vi "Read fit presets.vi"(0 "Config file in":T1, 11 "error in (no error)":errorcluster) -> (4 "Config file out":T1, 6 "Fit parameters":T3={"A"=0.572086, "S"=0.0835606, "M1"=140.286, "M2"=140.486}, 8 "Physical constants":T2={"T1e (s)"=0.03, "T1n (s)"=1500.0}, 10 "C":dbl, 14 "Key not found?":bool, 15 "error out":errorcluster)   [LabVIEW 2015]
uses:
  fit_parameters.ctl
  physical_constants.ctl
  <vilib>/Utility/config.llb/Config Data RefNum.ctl
  <vilib>/Utility/config.llb/Read Key (Double).vi
  <vilib>/Utility/config.llb/NI_LVConfig.lvlib
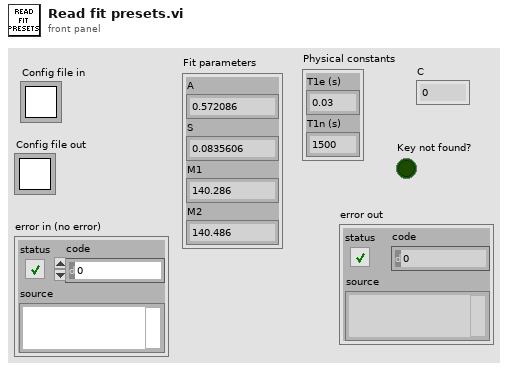
[diagram p1: front panel]
types:
  T1 = typedef "NI_LVConfig.lvlib/Config Data RefNum.ctl" = refnum<k1>
  T2 = typedef "physical_constants.ctl" = cluster{"T1e (s)":dbl, "T1n (s)":dbl}
  T3 = typedef "fit_parameters.ctl" = cluster{"A":dbl, "S":dbl, "M1":dbl, "M2":dbl}
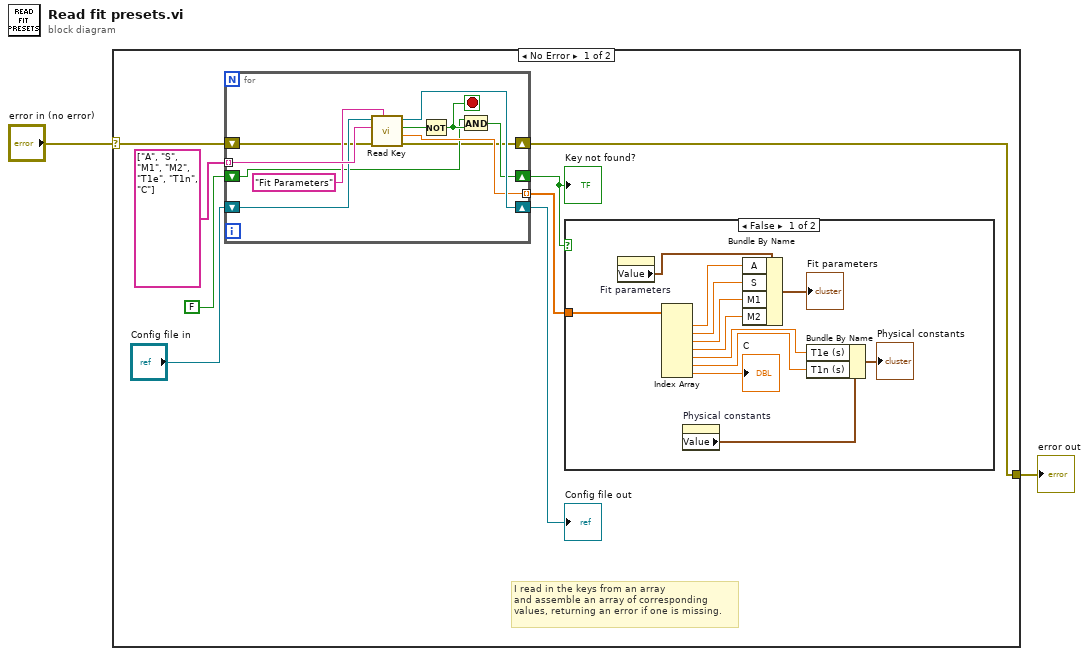
[diagram p0: block diagram]
diagram:
  n1 = case shown="No Error" "error in (no error)" {
    selector: "error in (no error)" -> [w4 w34]
    tunnel: [w3 w34] -> w1
    frame No Error {
      # "I read in the keys from an array\nand assemble an array of corresponding\nvalues, returning an error if one is missing."
      n2 = for {
        tunnel: string[] ["A", "S", "M1", "M2", "T1e", "T1n", "C"] -> [w33] mode=indexing
        shift-right: [w29] -> w5
        shift-left: "Config file in" -> [w30]
        tunnel: [w28] -> w9 mode=indexing
        shift-right: [w27] -> w7
        shift-left: FALSE -> [w25]
        shift-right: [w23] -> w3
        shift-left: w4 -> [w24]
        stop <- w26 stop-if-true
        n3 = call-poly <vilib>:"Read Key.vi"("section"="Fit Parameters", "error in (no error)"=w24, "key"=w33, "refnum"=w30) -> ("error out"=w23:errorcluster, "value"=w28:dbl, "found?"=w31:bool, "refnum out"=w29:T1)  [unwired: 4 in]
        n4 = Not(x=w31) -> (.not. x?=w26:bool)
        n5 = And(x=w25, y=w26) -> (x .and. y?=w27:bool)
      }
      "Key not found?" <- w7
      "Config file out" <- w5
      n6 = case shown="False" w7 {
        tunnel: w9 -> [w22 _]
        frame False {
          n7 = property on="Fit parameters" class="Clust (strict)"() -> ("Value"=w21:T3)  [unwired: 2 in, 2 out]
          n8 = Index Array(array=w22) -> (element #1=w19:dbl, element #2=w18:dbl, element #3=w17:dbl, element #4=w16:dbl, element #5=w15:dbl, element #6=w14:dbl, element #7=→"C":dbl)  [unwired: 7 in]
          n9 = property on="Physical constants" class="Clust (strict)"() -> ("Value"=w20:T2)  [unwired: 2 in, 2 out]
          n10 = Bundle By Name(cluster=w21, "A"=w19, "S"=w18, "M1"=w17, "M2"=w16) -> (→"Fit parameters":T3)
          n11 = Bundle By Name(cluster=w20, "T1e (s)"=w15, "T1n (s)"=w14) -> (→"Physical constants":T2)
        }
        frame True {
        }
      }
    }
    frame Error {
    }
  }
  "error out" <- w1
